vi "FPGA_ZAdjustment(NoSynchronizedDIO).vi"() -> ()   [LabVIEW 2014]
uses:
  <vilib>/rvi/Emulation/niFpgaGetClockAttributes.vi
  <vilib>/rvi/Emulation/niFpgaSctlEmulationGetInTimedLoop.vi
  <vilib>/rvi/Emulation/niFpgaEmulationReportErrorSimple.vi
  <vilib>/rvi/eio/common/nirviEmuTemplateMethod_errors.vi
  <vilib>/rvi/Emulation/niFpgaCriticalErrorInLSC.vi
  <vilib>/rvi/Emulation/niFpgaProcessEmulError.vi
  <vilib>/rvi/interface/RandomDataEmulation/niFpgaRandomDataHandleErrors.vi
  <vilib>/eio/EIONode/EIONode.xnode
  <vilib>/rvi/DataTransferAndStorage/Container/XNode/niFpgaContainer.xnode
  <vilib>/rvi/interface/RandomDataEmulation/nirviRandomDataFpgaReadWriteTemplate.vi
panel:
  out "Connector0/DIO0":bool
  out "Connector0/DIO2":bool
  out "ZRealTimePos":i16
  in  "stop":bool
  in  "ZOffset":i16
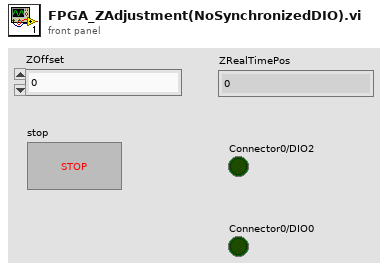
[diagram p1: front panel]
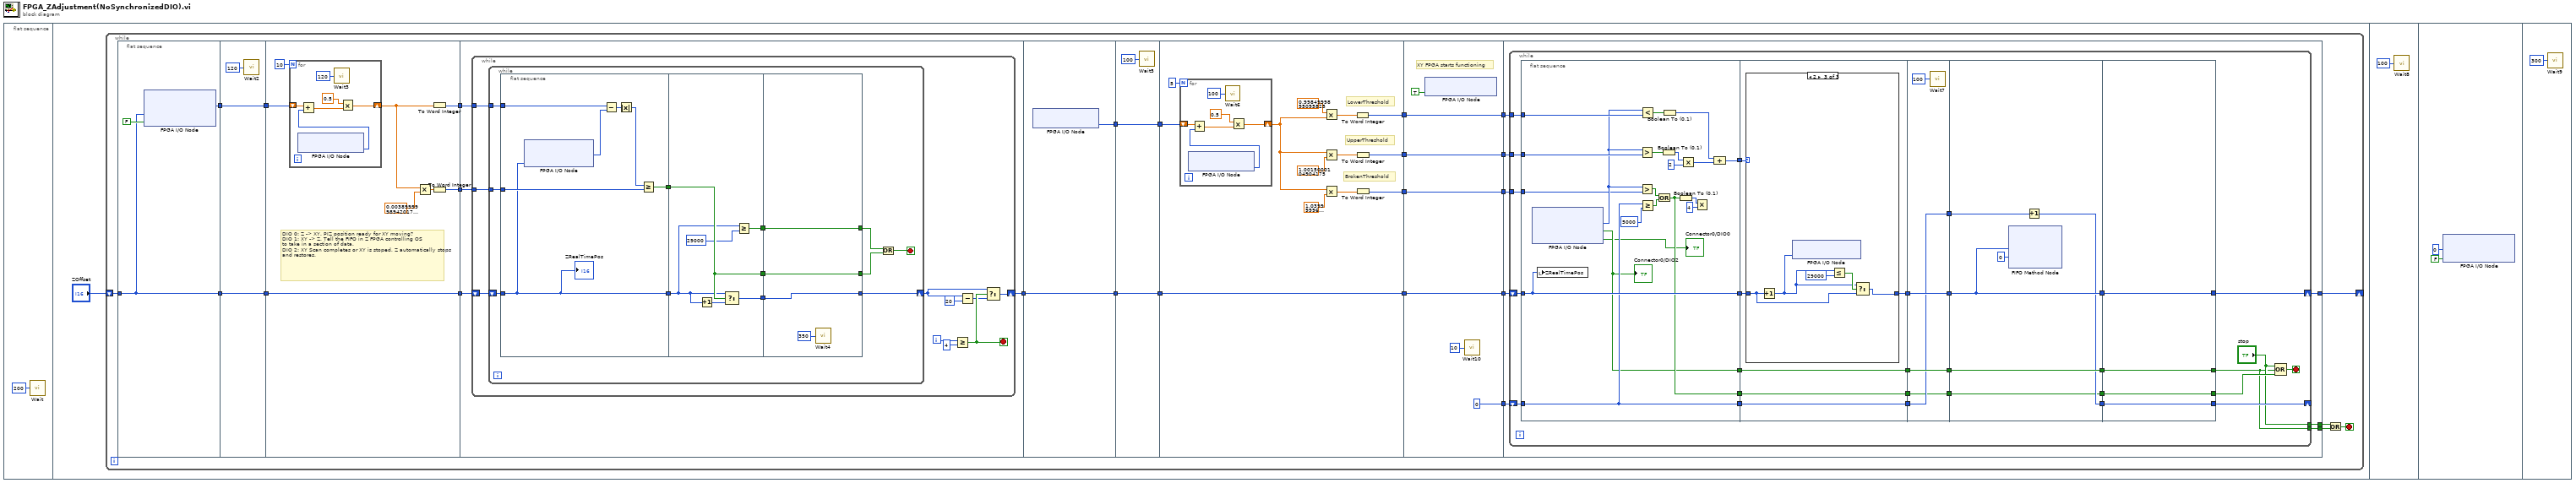
[diagram p0: block diagram]
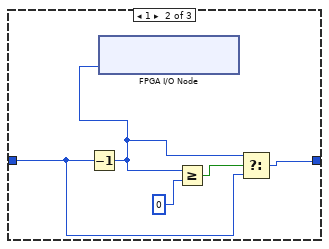
[diagram p3: hidden frame]
diagram:
  n1 = flat-sequence {
    frame #0 {
      n2 = call "Wait"("Count(uSec)"=u32 200) -> ()  [unwired: 1 out]
    }
    frame #1 {
      n3 = while {
        shift-right: [w7] -> _
        shift-left: "ZOffset" -> [w24]
        stop <- w5 stop-if-true
        n4 = flat-sequence {
          tunnel: [w31] -> w27
          tunnel: w24 -> [w29]
          tunnel: [w29] -> w22
          tunnel: [w33] -> w28
          tunnel: w27 -> [w33]
          tunnel: [w32] -> w23
          tunnel: w22 -> [w32]
          tunnel: w28 -> [w41]
          tunnel: [w37] -> w26
          tunnel: [w36] -> w25
          tunnel: w23 -> [w35]
          tunnel: [w35] -> w21
          tunnel: w26 -> [w52]
          tunnel: w25 -> [w51]
          tunnel: w21 -> [w50]
          tunnel: [w49] -> w20
          tunnel: w20 -> [w92]
          tunnel: [w93] -> w19
          tunnel: [w92] -> w10
          tunnel: w19 -> [w95]
          tunnel: [w95] -> w18
          tunnel: [w94] -> w11
          tunnel: w10 -> [w94]
          tunnel: w18 -> [w108]
          tunnel: [w100] -> w17
          tunnel: [w99] -> w15
          tunnel: [w98] -> w13
          tunnel: w11 -> [w97]
          tunnel: [w97] -> w8
          tunnel: w17 -> [w122]
          tunnel: [w122] -> w16
          tunnel: w15 -> [w121]
          tunnel: [w121] -> w14
          tunnel: w13 -> [w120]
          tunnel: [w120] -> w12
          tunnel: [w118] -> w9
          tunnel: w8 -> [w118]
          tunnel: [i16 0] -> w6
          tunnel: w16 -> [w130]
          tunnel: w14 -> [w129]
          tunnel: w12 -> [w128]
          tunnel: w9 -> [w127]
          tunnel: [w126] -> w7
          tunnel: w6 -> [w125]
          tunnel: [w124] -> w4
          tunnel: [w123] -> w3
          frame #0 {
            n5 = xnode "FPGA I/O Node"("Connector0/AO0"=w29, "Connector0/DIO0"=FALSE) -> ("Connector0/AI1"=w31:i16)  [unwired: 3 in, 3 out]
          }
          frame #1 {
            n6 = call "Wait2"("Count(uSec)"=u32 120) -> ()  [unwired: 1 out]
          }
          frame #2 {
            # "DIO 0: Z -> XY. PIZ position ready for XY moving?\nDIO 1: XY -> Z. Tell the FIFO in Z FPGA controlling OS\nto take in a section of data.\nDIO 2: XY Scan completes or XY is stoped, Z automatically stops and restores."
            n7 = for {
              N: 10 -> [_]
              shift-right: [w44] -> w39
              shift-left: w41 -> [w48]
              n8 = xnode "FPGA I/O Node"() -> ("Connector0/AI1"=w47:i16)  [unwired: 1 in, 1 out]
              n9 = Add(x=w48, y=w47) -> (x+y=w46:sgl)
              n10 = call "Wait3"("Count(uSec)"=u32 120) -> ()  [unwired: 1 out]
              n11 = Multiply(x=sgl 0.5, y=w46) -> (x*y=w44:sgl)
            }
            n12 = Multiply(x=w39, y=sgl 0.0039) -> (x*y=w38:sgl)
            n13 = To Word Integer(number=w39) -> (16bit integer=w37:i16)
            n14 = To Word Integer(number=w38) -> (16bit integer=w36:i16)
          }
          frame #3 {
            n15 = while {
              tunnel: w52 -> [w62]
              tunnel: w51 -> [w61]
              shift-right: [w58] -> w49
              shift-left: w50 -> [w60]
              i -> [w59]
              stop <- w57 stop-if-true
              n16 = while {
                tunnel: w62 -> [w74]
                tunnel: w61 -> [w73]
                shift-right: [w67] -> w56
                shift-left: w60 -> [w71]
                stop <- w65 stop-if-true
                n17 = flat-sequence {
                  tunnel: w74 -> [w81]
                  tunnel: w73 -> [w77]
                  tunnel: [w76] -> w72
                  tunnel: w71 -> [w75]
                  tunnel: [w75] -> w70
                  tunnel: w72 -> [w85]
                  tunnel: w70 -> [w84]
                  tunnel: [w86] -> w69
                  tunnel: [w85] -> w68
                  tunnel: [w82] -> w66
                  tunnel: w69 -> [w89]
                  tunnel: w68 -> [w90]
                  tunnel: [w90] -> w63
                  tunnel: [w89] -> w67
                  tunnel: [w88] -> w64
                  tunnel: w66 -> [w88]
                  frame #0 {
                    n18 = xnode "FPGA I/O Node"("Connector0/AO0"=w75) -> ("Connector0/AI1"=w80:i16)  [unwired: 2 in, 2 out]
                    n19 = Subtract(x=w81, y=w80) -> (x-y=w79:i16)
                    n20 = Absolute Value(x=w79) -> (abs(x)=w78:i16)
                    n21 = Greater Or Equal?(x=w78, y=w77) -> (x >= y?=w76:bool)
                    "ZRealTimePos" <- w75
                  }
                  frame #1 {
                    n22 = Increment(x=w84) -> (x+1=w87:i16)
                    n23 = Select(t=w84, s=w85, f=w87) -> (s? t:f=w86:i16)
                    n24 = Greater Or Equal?(x=w84, y=i16 29000) -> (x >= y?=w82:bool)
                  }
                  frame #2 {
                    n25 = call "Wait4"("Count(uSec)"=u32 350) -> ()  [unwired: 1 out]
                  }
                }
                n26 = Or(x=w64, y=w63) -> (x .or. y?=w65:bool)
              }
              n27 = Greater Or Equal?(x=w59, y=4) -> (x >= y?=w57:bool)
              n28 = Subtract(x=w56, y=i16 20) -> (x-y=w54:i16)
              n29 = Select(t=w56, s=w57, f=w54) -> (s? t:f=w58:i16)
            }
          }
          frame #4 {
            n30 = xnode "FPGA I/O Node"() -> ("Connector0/AI1"=w93:i16)  [unwired: 1 in, 1 out]
          }
          frame #5 {
            n31 = call "Wait5"("Count(uSec)"=u32 100) -> ()  [unwired: 1 out]
          }
          frame #6 {
            # "BrokenThreshold"
            # "UpperThreshold"
            # "LowerThreshold"
            n32 = for {
              N: 5 -> [_]
              shift-right: [w111] -> w101
              shift-left: w108 -> [w115]
              n33 = xnode "FPGA I/O Node"() -> ("Connector0/AI1"=w114:i16)  [unwired: 1 in, 1 out]
              n34 = Add(x=w115, y=w114) -> (x+y=w113:sgl)
              n35 = call "Wait6"("Count(uSec)"=u32 100) -> ()  [unwired: 1 out]
              n36 = Multiply(x=sgl 0.5, y=w113) -> (x*y=w111:sgl)
            }
            n37 = Multiply(x=sgl 0.9985 ("y"), y=w101) -> (x*y=w105:sgl)
            n38 = Multiply(x=w101, y=sgl 1.0015) -> (x*y=w104:sgl)
            n39 = Multiply(x=w101, y=sgl 1.04) -> (x*y=w102:sgl)
            n40 = To Word Integer(number=w105) -> (16bit integer=w100:i16)
            n41 = To Word Integer(number=w104) -> (16bit integer=w99:i16)
            n42 = To Word Integer(number=w102) -> (16bit integer=w98:i16)
          }
          frame #7 {
            # "XY FPGA starts functioning"
            n43 = xnode "FPGA I/O Node"("Connector0/DIO0"=TRUE) -> ()  [unwired: 1 in, 1 out]
            n44 = call "Wait10"("Count(uSec)"=u32 10) -> ()  [unwired: 1 out]
          }
          frame #8 {
            n45 = while {
              tunnel: w130 -> [w158]
              tunnel: w129 -> [w157]
              tunnel: w128 -> [w156]
              shift-right: [w147] -> w126
              shift-left: w127 -> [w155]
              shift-right: [w142] -> _
              shift-left: w125 -> [w146]
              tunnel: ["stop"] -> w124
              tunnel: [w135] -> w123
              stop <- w138 stop-if-true
              n46 = flat-sequence {
                tunnel: w158 -> [w179]
                tunnel: w157 -> [w178]
                tunnel: w156 -> [w176]
                tunnel: w155 -> [w166]
                tunnel: [w167] -> w154
                tunnel: [w160] -> w153
                tunnel: [w166] -> w150
                tunnel: w146 -> [w163]
                tunnel: [w163] -> w143
                tunnel: [w161] -> w141
                tunnel: w154 -> [w185]
                tunnel: w153 -> [w184]
                tunnel: [w184] -> w151
                tunnel: w150 -> [w183]
                tunnel: [w182] -> w149
                tunnel: [w181] -> w144
                tunnel: w143 -> [w181]
                tunnel: w141 -> [w180]
                tunnel: [w180] -> w140
                tunnel: [w200] -> w152
                tunnel: w151 -> [w200]
                tunnel: w149 -> [w199]
                tunnel: [w199] -> w148
                tunnel: [w198] -> w145
                tunnel: w144 -> [w198]
                tunnel: w140 -> [w197]
                tunnel: [w197] -> w139
                tunnel: w152 -> [w207]
                tunnel: w148 -> [w206]
                tunnel: w145 -> [w205]
                tunnel: w139 -> [w203]
                tunnel: [w207] -> w134
                tunnel: [w206] -> w133
                tunnel: [w204] -> w132
                tunnel: [w203] -> w131
                tunnel: [w208] -> w137
                tunnel: [w209] -> w142
                tunnel: [w210] -> w147
                tunnel: [w211] -> w135
                tunnel: w134 -> [w211]
                tunnel: w133 -> [w210]
                tunnel: w132 -> [w209]
                tunnel: w131 -> [w208]
                frame #0 {
                  n47 = xnode "FPGA I/O Node"() -> ("Connector0/AI1"=w177:i16, "Connector0/DIO2"=w160:bool, "Connector0/DIO0"=→"Connector0/DIO0":bool)  [unwired: 3 in, 3 out]
                  "Connector0/DIO2" <- w160
                  n48 = local write "ZRealTimePos"(w166) -> ()
                  n49 = Greater?(x=w177, y=w178) -> (0:w174:bool)
                  n50 = Greater?(x=w177, y=w176) -> (0:w165:bool)
                  n51 = Less?(x=w177, y=w179) -> (x < y?=w175:bool)
                  n52 = Greater Or Equal?(x=w163, y=i16 5000) -> (x >= y?=w164:bool)
                  n53 = Or(x=w165, y=w164) -> (x .or. y?=w161:bool)
                  n54 = Boolean To (0,1)(Boolean=w174) -> (0, 1=w173:i16)
                  n55 = Boolean To (0,1)(Boolean=w175) -> (0, 1=w169:i16)
                  n56 = Boolean To (0,1)(Boolean=w161) -> (0, 1=w171:i16)
                  n57 = Multiply(x=w173, y=i16 2) -> (x*y=w168:i16)
                  n58 = Multiply(x=w171, y=i16 4) -> ()  [unwired: 1 out]
                  n59 = Compound Arithmetic op=unknown(w169, w168) -> (w167:i16)
                }
                frame #1 {
                  n60 = case shown="2" w185 {
                    tunnel: w183 -> [w186 w187 w192]
                    tunnel: [w186 w189 w194] -> w182
                    frame 0, Default {
                    }
                    frame 1 {
                      n61 = Decrement(x=w187) -> (x-1=w188:i16)
                      n62 = xnode "FPGA I/O Node"("Connector0/AO0"=w188) -> ()  [unwired: 1 in, 1 out]
                      n63 = Greater Or Equal?(x=w188, y=i16 0) -> (x >= y?=w191:bool)
                      n64 = Select(t=w188, s=w191, f=w187) -> (s? t:f=w189:i16)
                    }
                    frame 2 {
                      n65 = Increment(x=w192) -> (x+1=w193:i16)
                      n66 = xnode "FPGA I/O Node"("Connector0/AO0"=w193) -> ()  [unwired: 1 in, 1 out]
                      n67 = Less Or Equal?(x=w193, y=i16 29000) -> (x <= y?=w195:bool)
                      n68 = Select(t=w193, s=w195, f=w192) -> (s? t:f=w194:i16)
                    }
                  }
                }
                frame #2 {
                  n69 = call "Wait7"("Count(uSec)"=u32 100) -> ()  [unwired: 1 out]
                }
                frame #3 {
                  n70 = xnode ("FIFO Method Node")("Element"=w206, "Timeout"=0) -> ()  [unwired: 1 in, 2 out]
                  n71 = Increment(x=w205) -> (x+1=w204:i16)
                }
                frame #4 {
                }
              }
              n72 = Compound Arithmetic op=OR("stop", w135, w137) -> (w138:bool)
            }
          }
        }
        n73 = Or(x=w4, y=w3) -> (x .or. y?=w5:bool)
      }
    }
    frame #2 {
      n74 = call "Wait8"("Count(uSec)"=u32 100) -> ()  [unwired: 1 out]
    }
    frame #3 {
      n75 = xnode "FPGA I/O Node"("Connector0/AO0"=i16 0, "Connector0/DIO0"=FALSE) -> ()  [unwired: 2 in, 2 out]
    }
    frame #4 {
      n76 = call "Wait9"("Count(uSec)"=u32 300) -> ()  [unwired: 1 out]
    }
  }
